vi "SubVI_Example_Get_AutoFeatures_Software_Shutter.vi"(8 "error in (no error)":errorcluster caption="Fehler (Eingang, kein Fehler)", 11 ".NET (Reference)":refnum<k24>) -> (0 "error out":errorcluster caption="Fehler (Ausgang)", 2 "Enabled":bool, 3 "Supported":bool)   [LabVIEW 2017]
uses:
  C:/Users/George Sirinakis/Desktop/Microscope Control/Device Library/Cameras/IDS/IDS LabView Examples/LabVIEW/ueye.NET/uEyeDotNet.dll
  uEyeDotNet.dll
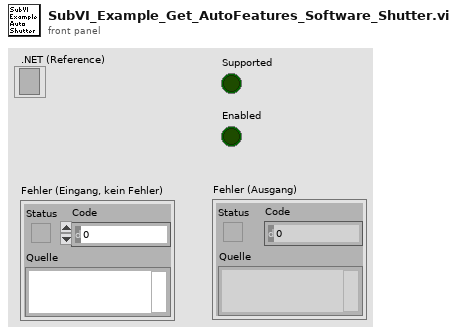
[diagram p1: front panel]
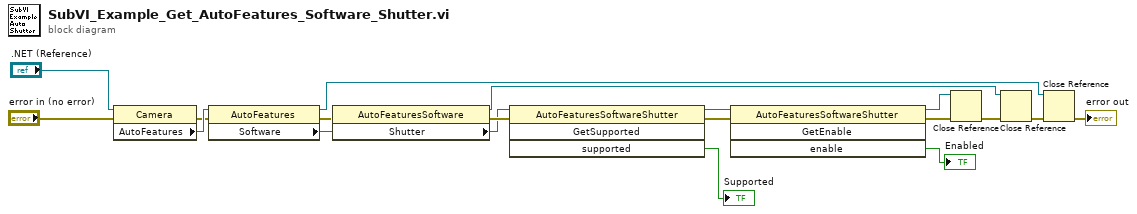
[diagram p0: block diagram]
diagram:
  n1 = property class="Camera"(reference=".NET (Reference)", error in="error in (no error)") -> (error out=w18:errorcluster, "AutoFeatures"=w19:refnum<k24>)  [unwired: 1 out]
  n2 = property class="AutoFeatures"(reference=w19, error in=w18) -> (reference out=w14:refnum<k24>, error out=w16:errorcluster, "Software"=w17:refnum<k24>)
  n3 = property class="AutoFeaturesSoftware"(reference=w17, error in=w16) -> (reference out=w15:refnum<k24>, error out=w11:errorcluster, "Shutter"=w6:refnum<k24>)
  n4 = invoke class="AutoFeaturesSoftwareShutter" method="GetSupported"(reference=w6, error in=w11) -> (reference out=w9:refnum<k24>, error out=w10:errorcluster, "supported"=→"Supported":bool)  [unwired: 2 in, 1 out]
  n5 = invoke class="AutoFeaturesSoftwareShutter" method="GetEnable"(reference=w9, error in=w10) -> (reference out=w8:refnum<k24>, error out=w7:errorcluster, "enable"=→"Enabled":bool)  [unwired: 2 in, 1 out]
  n6 = Close Reference(reference=w8, error in (no error)=w7) -> (error out=w12:errorcluster)
  n7 = Close Reference(reference=w15, error in (no error)=w12) -> (error out=w13:errorcluster)
  n8 = Close Reference(reference=w14, error in (no error)=w13) -> (error out=→"error out":errorcluster)
